vi "Severity - rank compare.vi"(8 "error in (no error)":errorcluster) -> (0 "error out":errorcluster)   [LabVIEW 2026, in "Tests.lvlib"]
doc: "Description: Unit test (Caraya). Verifies RankCompare gates by Severity rank: a more-severe level passes its threshold, a less-severe level is dropped, the equal-rank boundary passes, OFF disables all logging, and ALL passes every level (SRS-LMBR-005, 006). Pure, no actors or I/O."
uses:
  Tests.lvlib
  src/TypeDefs/Severity.ctl
  <vilib>/addons/_JKI Toolkits/Caraya/classes/Assert/Assert True.vi
  <vilib>/addons/_JKI Toolkits/Caraya/classes/Assert/Assert False.vi
  src/Lumberjack.lvlib
  <vilib>/addons/_JKI Toolkits/Caraya/classes/Assert/Assert.lvclass
  <vilib>/addons/_JKI Toolkits/Caraya/classes/Test/Test.lvclass
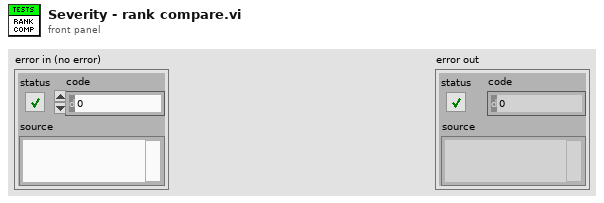
[diagram p1: front panel]
types:
  T1 = typedef "Lumberjack.lvlib/Severity.ctl" = enum16{"OFF", "FATAL", "ERROR", "WARN", "INFO", "DEBUG", "TRACE", "ALL"}
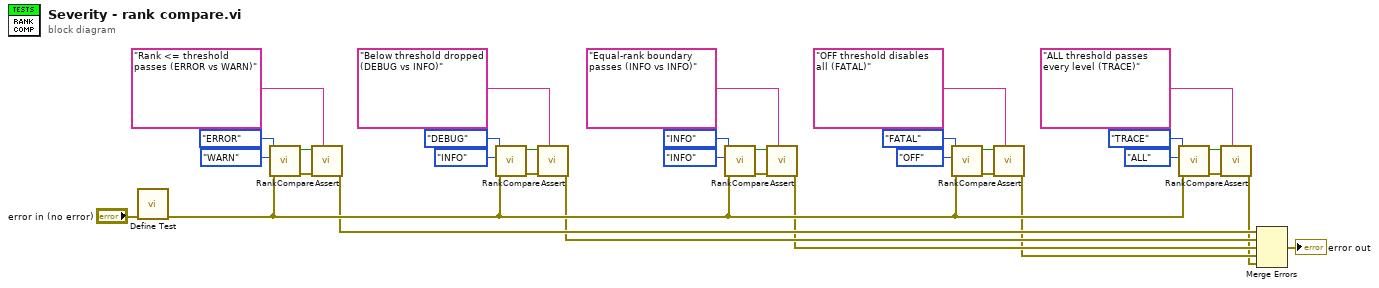
[diagram p0: block diagram]
diagram:
  n1 = call <vilib>:"Define Test.vi"("error in (no error)"="error in (no error)") -> ("error out"=w8:errorcluster)  [unwired: 9 in, 1 out]
  n2 = call "RankCompare.vi"("error in (no error)"=w8, "Threshold"=Severity."WARN" ("Level"), "Level"=Severity."ERROR") -> ("error out"=w31:errorcluster, "Passes"=w30:bool)  [unwired: 7 in]
  n3 = call-poly <vilib>:"Assert.vi"("Label"="Rank <= threshold passes (ERROR vs WARN)", "error in (no error)"=w31, "True?"=w30) -> ("error out"=w7:errorcluster)  [unwired: 7 in, 1 out]
  n4 = call "RankCompare.vi"("error in (no error)"=w8, "Threshold"=Severity."INFO" ("Level"), "Level"=Severity."DEBUG") -> ("error out"=w26:errorcluster, "Passes"=w25:bool)  [unwired: 7 in]
  n5 = call-poly <vilib>:"Assert.vi"("Label"="Below threshold dropped (DEBUG vs INFO)", "error in (no error)"=w26, "False?"=w25) -> ("error out"=w6:errorcluster)  [unwired: 7 in, 1 out]
  n6 = call "RankCompare.vi"("error in (no error)"=w8, "Threshold"=Severity."INFO" ("Level"), "Level"=Severity."INFO") -> ("error out"=w21:errorcluster, "Passes"=w20:bool)  [unwired: 7 in]
  n7 = call-poly <vilib>:"Assert.vi"("Label"="Equal-rank boundary passes (INFO vs INFO)", "error in (no error)"=w21, "True?"=w20) -> ("error out"=w5:errorcluster)  [unwired: 7 in, 1 out]
  n8 = call "RankCompare.vi"("error in (no error)"=w8, "Threshold"=Severity."OFF" ("Level"), "Level"=Severity."FATAL") -> ("error out"=w16:errorcluster, "Passes"=w15:bool)  [unwired: 7 in]
  n9 = call-poly <vilib>:"Assert.vi"("Label"="OFF threshold disables all (FATAL)", "error in (no error)"=w16, "False?"=w15) -> ("error out"=w4:errorcluster)  [unwired: 7 in, 1 out]
  n10 = call "RankCompare.vi"("error in (no error)"=w8, "Threshold"=Severity."ALL" ("Level"), "Level"=Severity."TRACE") -> ("error out"=w11:errorcluster, "Passes"=w10:bool)  [unwired: 7 in]
  n11 = call-poly <vilib>:"Assert.vi"("Label"="ALL threshold passes every level (TRACE)", "error in (no error)"=w11, "True?"=w10) -> ("error out"=w3:errorcluster)  [unwired: 7 in, 1 out]
  n12 = Merge Errors(w7, w6, w5, w4, w3) -> (→"error out":errorcluster)
